vi "Create Method VIs.vi"(7 "Template Class":refnum<vi>, 9 "Methods":T2[](array[typedef]), 10 "Class Param Writer":refnum<class "Abstract Param Writer.lvclass">, 11 "Class":refnum<vi>) -> (2 "Method Ref Map":T1, 3 "Class Dup":refnum<vi>)   [LabVIEW 2013]
uses:
  Data Structures/JSON/Method.ctl
  Data Structures/JSON/Param.ctl
  <userlib>/ICON Technologies/ICON Maps/lvlib/Map.ctl
  Param Writers/Abstract Param Writer/Abstract Param Writer.lvclass
  <vilib>/Utility/traverseref.llb/TRef TravTarget.ctl
  Data Structures/DLL Parameter Info.ctl
  Icons and Wires/Icon Template.ctl
  Param Writers/TypeConv/Action.ctl
  <userlib>/ICON Technologies/ICON Maps/lvlib/_Polymorphic Instances/Map_Insert_Variant.vi
  <vilib>/regexp/Match Regular Expression.xnode
  <vilib>/Utility/traverseref.llb/VI Scripting - Traverse.lvlib
  <userlib>/ICON Technologies/ICON Maps/ICON Maps.lvlib
  <vilib>/LabVIEW Icon API/LabVIEW Icon API.lvlib
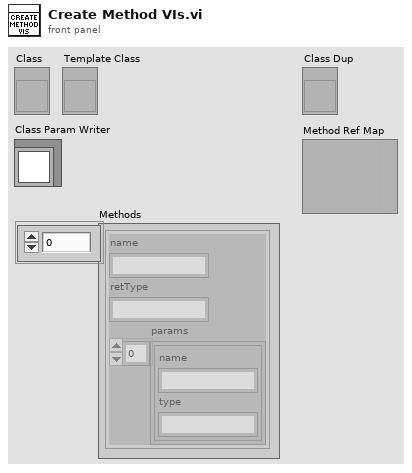
[diagram p1: front panel]
types:
  T1 = typedef "ICON Maps.lvlib/Map.ctl" = variant
  T2 = typedef "Method.ctl" = cluster{"name":string, "retType":string, "params":T3[]}
  T3 = typedef "Param.ctl" = cluster{"name":string, "type":string}
  T4 = typedef "TRef TravTarget.ctl" = enum16{"FP", "BD", "Other"}
  T5 = typedef "Icon Template.ctl" = enum16{"1-Segment, Light", "1-Segment, Dark", "2-Segment, Light", "2-Segment, Dark"}
  T6 = typedef "Action.ctl" = enum16{"Register Type", "Obtain Writer"}
  T7 = typedef "DLL Parameter Info.ctl" = cluster{"Parameter Name":string, "Num Dimensions":i32, "Parameter Type":enum16{"Numeric", "Array", "String", "Waveform", "Digital Waveform", "Digital Table", "ActiveX", "Any", "Instance Data Pointer", "Void"}, "Numeric Type":enum16{"I8", "I16", "I32", "I64", "U8", "U16", "U32", "U64", "SGL", "DBL", "PTR INT", "PTR UINT"}, "Param Passing":enum16{"By Value", "Pointer To Value"}, "Array Passing":enum16{"Array Data Pointer", "Array Handle", "Array Handle Pointer"}, "String Passing":enum16{"C String Pointer", "Pascal String Pointer", "String Handle", "String Handle Pointer"}, "Adapt Format":enum16{"By Value", "Pointer To Value"}, "ActiveX Types":enum16{"ActiveX Variant Pointer", "IDispatch* Pointer", "IUnknown* Pointer"}, "Const (unused)":bool, "Minimum Size":string}
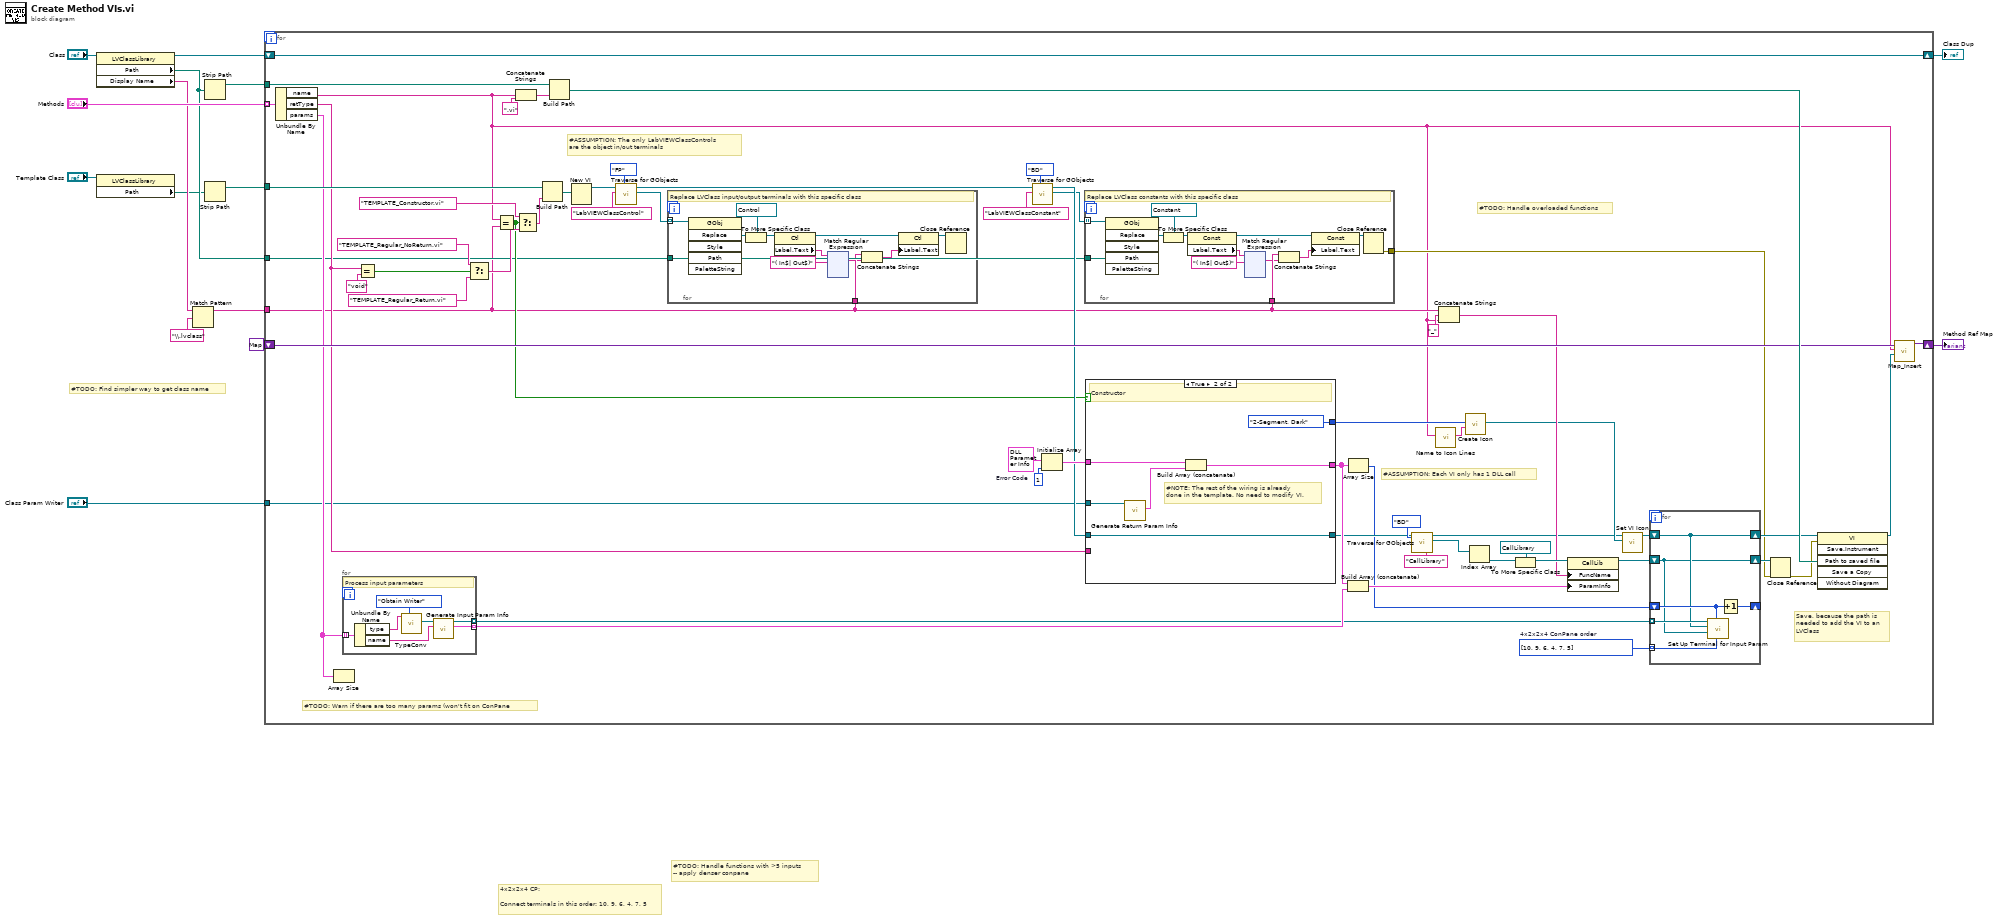
[diagram p0: block diagram]
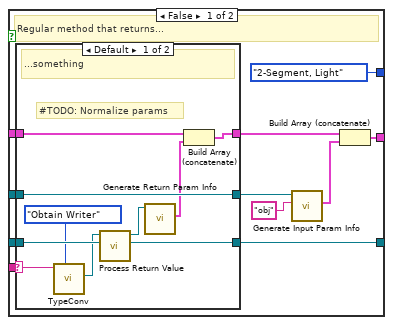
[diagram p2: hidden frame]
diagram:
  # "#TODO: Handle functions with >5 inputs\n-- apply denser conpane"
  # "4x2x2x4 CP:\n\nConnect terminals in this order: 10, 9, 6, 4, 7, 5"
  # "#TODO: Find simpler way to get class name"
  n1 = property class="LVClassLibrary"(reference="Class") -> (reference out=w7:refnum<vi>, "Path"=w12:path, "Display Name"=w10:string)  [unwired: 1 in, 1 out]
  n2 = property class="LVClassLibrary"(reference="Template Class") -> ("Path"=w3:path)  [unwired: 1 in, 2 out]
  n3 = Match Pattern(string=w10, regular expression="\\.lvclass") -> (before substring=w9:string)  [unwired: 1 in, 3 out]
  n4 = Strip Path(path=w12) -> (stripped path=w14:path)  [unwired: 1 out]
  n5 = Strip Path(path=w3) -> (stripped path=w2:path)  [unwired: 1 out]
  n6 = for {
    tunnel: "Methods" -> [w77] mode=indexing
    tunnel: w2 -> [w50]
    tunnel: w14 -> [w75]
    shift-right: [w73] -> w15
    shift-left: w7 -> [w73]
    tunnel: w12 -> [w26]
    tunnel: w9 -> [w24]
    shift-right: [w66] -> w5
    shift-left: T1 variant ("Map Out") -> [w65]
    tunnel: "Class Param Writer" -> [w22]
    w29 = i32[] [10, 9, 6, 4, 7, 5]  # 4x2x2x4 ConPane order
    w42 = T7 {"Parameter Name"="errorCode", "Num Dimensions"=1, "Parameter Type"=enum."Numeric", "Numeric Type"=enum."I32", "Param Passing"=enum."By Value", "Array Passing"=enum."Array Data Pointer", "String Passing"=enum."C String Pointer", "Adapt Format"=enum."By Value", "ActiveX Types"=enum."ActiveX Variant Pointer", "Const (unused)"=FALSE, "Minimum Size"=""}  # Error Code
    # "#TODO: Warn if there are too many params (won't fit on ConPane"
    # "#TODO: Handle overloaded functions"
    # "Save, because the path is\nneeded to add the VI to an\nLVClass"
    # "#ASSUMPTION: Each VI only has 1 DLL call"
    # "#ASSUMPTION: The only LabVIEWClassControls\nare the object in/out terminals"
    n7 = Unbundle By Name(w77) -> ("name"=w20:string, "retType"=w44:string, "params"=w32:T3[])
    n8 = Array Size(array=w32) -> ()  [unwired: 1 out]
    n9 = for {
      tunnel: w32 -> [w247] mode=indexing
      tunnel: [w245] -> w36 mode=indexing
      tunnel: [w244] -> w33 mode=indexing
      # "Process input parameters"
      n10 = Unbundle By Name(w247) -> ("type"=w242:string, "name"=w246:string)
      n11 = call "TypeConv.vi"("Action"=Action."Obtain Writer", "Type Name"=w242) -> ("Param Writer"=w241:refnum<class "Abstract Param Writer.lvclass">)  [unwired: 9 in]
      n12 = call-dynamic "Generate Input Param Info.vi"("Param Name"=w246, "Abstract Param Writer in"=w241) -> ("Param Info"=w245:T7, "Abstract Param Writer out"=w244:refnum<class "Abstract Param Writer.lvclass">)  [unwired: 8 in]
    }
    n13 = Equal?(x=w44, y="void") -> (x = y?=w28:bool)
    n14 = Select(t="TEMPLATE_Regular_NoReturn.vi" ("string"), s=w28, f="TEMPLATE_Regular_Return.vi" ("string")) -> (s? t:f=w45:string)
    n15 = Equal?(x=w20, y=w24) -> (x = y?=w27:bool)
    n16 = Concatenate Strings(w20, ".vi" ("string")) -> (w74:string)
    n17 = Select(t="TEMPLATE_Constructor.vi" ("string"), s=w27, f=w45) -> (s? t:f=w51:string)
    n18 = Build Path(base path=w50, name or relative path=w51) -> (appended path=w49:path)
    n19 = Build Path(base path=w75, name or relative path=w74) -> (appended path=w68:path)
    n20 = New VI(10:w49) -> (3:w72:refnum<vi>)  [unwired: 6 in, 1 out]
    n21 = call <vilib>:"Traverse for GObjects.vi"("Traverse Target"=TRef_TravTarget."FP", "Class Name"="LabVIEWClassControl", "VI Refnum"=w72) -> ("References"=w70:refnum<vi>[], "dup VI Refnum"=w55:refnum<vi>)  [unwired: 5 in, 2 out]
    n22 = for {
      tunnel: w70 -> [w258] mode=indexing
      tunnel: w26 -> [w257]
      tunnel: w24 -> [w259]
      # "Replace LVClass input/output terminals with this specific class"
      n23 = invoke class="GObj" method="Replace"(reference=w258, "Path"=w257) -> ("Replace"=w255:refnum<vi>)  [unwired: 4 in, 5 out]
      n24 = To More Specific Class(target class=refnum<vi> refnum ("Replace"), reference=w255) -> (specific class reference=w254:refnum<vi>)  [unwired: 1 in, 1 out]
      n25 = property class="Ctl"(reference=w254) -> (reference out=w253:refnum<vi>, "Label.Text"=w251:string)  [unwired: 1 in, 1 out]
      n26 = xnode "Match Regular Expression"("input string"=w251, "regular expression"="( In$| Out$)") -> ("whole match"=w249:string)  [unwired: 4 in, 4 out]
      n27 = Concatenate Strings(w259, w249) -> (w248:string)
      n28 = property class="Ctl"(reference=w253, "Label.Text"=w248) -> (reference out=w252:refnum<vi>)  [unwired: 1 in, 1 out]
      n29 = Close Reference(reference=w252) -> ()  [unwired: 1 in, 1 out]
    }
    n30 = call <vilib>:"Traverse for GObjects.vi"("Traverse Target"=TRef_TravTarget."BD", "Class Name"="LabVIEWClassConstant", "VI Refnum"=w55) -> ("References"=w23:refnum<vi>[], "dup VI Refnum"=w38:refnum<vi>)  [unwired: 5 in, 2 out]
    n31 = Initialize Array(w42, 1 ("dimension size")) -> (w41:T7[])
    n32 = for {
      tunnel: w23 -> [w89] mode=indexing
      tunnel: w26 -> [w88]
      tunnel: w24 -> [w90]
      tunnel: [w78] -> w25
      # "Replace LVClass constants with this specific class"
      n33 = invoke class="GObj" method="Replace"(reference=w89, "Path"=w88) -> ("Replace"=w86:refnum<vi>)  [unwired: 4 in, 5 out]
      n34 = To More Specific Class(target class=refnum<vi> refnum ("Replace"), reference=w86) -> (specific class reference=w85:refnum<vi>)  [unwired: 1 in, 1 out]
      n35 = property class="Const"(reference=w85) -> (reference out=w84:refnum<vi>, "Label.Text"=w82:string)  [unwired: 1 in, 1 out]
      n36 = xnode "Match Regular Expression"("input string"=w82, "regular expression"="( In$| Out$)") -> ("whole match"=w80:string)  [unwired: 4 in, 4 out]
      n37 = Concatenate Strings(w90, w80) -> (w79:string)
      n38 = property class="Const"(reference=w84, "Label.Text"=w79) -> (reference out=w83:refnum<vi>)  [unwired: 1 in, 1 out]
      n39 = Close Reference(reference=w83) -> (error out=w78:errorcluster)  [unwired: 1 in]
    }
    n40 = case shown="True" w27 {
      tunnel: w44 -> [w210 _]
      tunnel: w41 -> [w215 w233]
      tunnel: [w213 w232] -> w39
      tunnel: w38 -> [w212 w234]
      tunnel: [w211 w234] -> w37
      tunnel: w22 -> [w208 w230]
      tunnel: [Icon_Template."2-Segment, Light" ("Icon Template") Icon_Template."2-Segment, Dark" ("Icon Template")] -> w21
      frame False {
        # "Regular method that returns..."
        n41 = case shown="Default" w210 {
          selector: w210 -> [w219 _]
          tunnel: w215 -> [w223 w228]
          tunnel: w212 -> [w225 w227]
          tunnel: [w224 w228] -> w214
          tunnel: [w222 w227] -> w211
          tunnel: [w218 w226] -> w209
          tunnel: w208 -> [w218 w226]
          frame Default {
            # "#TODO: Normalize params"
            # "...something"
            n42 = call "TypeConv.vi"("Action"=Action."Obtain Writer", "Type Name"=w219) -> ("Param Writer"=w220:refnum<class "Abstract Param Writer.lvclass">)  [unwired: 9 in]
            n43 = call-dynamic "Process Return Value.vi"("Method VI"=w225, "Abstract Param Writer in"=w220) -> ("Modified Proto Method  VI"=w222:refnum<vi>, "Abstract Param Writer out"=w217:refnum<class "Abstract Param Writer.lvclass">)  [unwired: 8 in]
            n44 = call-dynamic "Generate Return Param Info.vi"("Abstract Param Writer in"=w217) -> ("Param Info"=w216:T7)  [unwired: 9 in, 1 out]
            n45 = Build Array (concatenate)(w223, w216) -> (w224:T7[])
          }
          frame "void" {
            # "...nothing"
          }
        }
        n46 = call-dynamic "Generate Input Param Info.vi"("Param Name"="obj", "Abstract Param Writer in"=w209) -> ("Param Info"=w207:T7)  [unwired: 8 in, 1 out]
        n47 = Build Array (concatenate)(w214, w207) -> (w213:T7[])
      }
      frame True {
        # "#NOTE: The rest of the wiring is already\ndone in the template. No need to modify VI."
        # "Constructor"
        n48 = call-dynamic "Generate Return Param Info.vi"("Abstract Param Writer in"=w230) -> ("Param Info"=w231:T7)  [unwired: 9 in, 1 out]
        n49 = Build Array (concatenate)(w233, w231) -> (w232:T7[])
      }
    }
    n50 = Build Array (concatenate)(w39, w36) -> (w40:T7[])
    n51 = Array Size(array=w39) -> (size(s)=w31:i32)
    n52 = call <vilib>:"Traverse for GObjects.vi"("Traverse Target"=TRef_TravTarget."BD", "Class Name"="CallLibrary", "VI Refnum"=w37) -> ("References"=w60:refnum<vi>[], "dup VI Refnum"=w17:refnum<vi>)  [unwired: 5 in, 2 out]
    n53 = call "Name to Icon Lines.vi"("Name"=w20) -> ("Lines"=w19:string[])  [unwired: 10 in]
    n54 = Concatenate Strings(w24, "_" ("string"), w20) -> (w57:string)
    n55 = call "Create Icon.vi"("Text"=w19, "Icon Template"=w21) -> ("Icon"=w18:refnum<class "Icon.lvclass">)  [unwired: 9 in]
    n56 = Index Array(array=w60) -> (element=w59:refnum<vi>)  [unwired: 1 in]
    n57 = To More Specific Class(target class=refnum<vi> refnum ("Replace"), reference=w59) -> (specific class reference=w58:refnum<vi>)  [unwired: 1 in, 1 out]
    n58 = property class="CallLib"(reference=w58, "FuncName"=w57, "ParamInfo"=w40) -> (reference out=w30:refnum<vi>)  [unwired: 1 in, 1 out]
    n59 = call <vilib>:"Set VI Icon.vi"("Icon"=w18, "VI Refnum in"=w17) -> ("VI Refnum out"=w16:refnum<vi>)  [unwired: 8 in, 1 out]
    n60 = for {
      shift-right: [w237] -> w34
      shift-left: w16 -> [w237]
      shift-right: [w236] -> w35
      shift-left: w30 -> [w236]
      tunnel: w33 -> [w240] mode=indexing
      shift-right: [w238] -> _
      shift-left: w31 -> [w239]
      tunnel: w29 -> [w235] mode=indexing
      n61 = call-dynamic "Set Up Terminal for Input Param.vi"("ConPane Terminal Index"=w235, "CallLibrary Terminal Index"=w239, "CalllLibrary Ref"=w236, "VI Ref"=w237, "Abstract Param Writer in"=w240) -> ()  [unwired: 6 in, 1 out]
      n62 = Increment(x=w239) -> (x+1=w238:i32)
    }
    n63 = Close Reference(reference=w35, error in (no error)=w25) -> (error out=w56:errorcluster)
    n64 = invoke class="VI" method="Save.Instrument"(reference=w34, error in=w56, "Path to saved file"=w68) -> (reference out=w67:refnum<vi>)  [unwired: 3 in, 5 out]
    n65 = call-poly <userlib>:"Map_Insert.vi"("Value"=w67, "Key"=w20, "Map In"=w65) -> ("Map Out"=w66:T1)  [unwired: 8 in]
  }
  "Class Dup" <- w15
  "Method Ref Map" <- w5
